vi "AddtoCurveList.vi"(8 "error in (no error)":errorcluster caption="entrée d'erreur (pas d'erreur)", 11 "Interface en entrée":refnum<class "Interface.lvclass"> caption="DNL_LabVIEW Object in") -> (0 "error out":errorcluster caption="sortie d'erreur", 3 "Interface en sortie":refnum<class "Interface.lvclass"> caption="DNL_LabVIEW Object out")   [LabVIEW 2010, in "Interface.lvclass"]
uses:
  Interface.lvclass
  Interface.lvclass/Interface.ctl
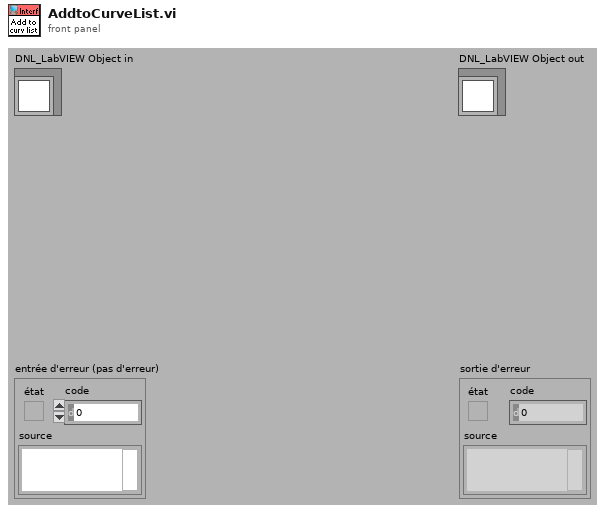
[diagram p1: front panel]
types:
  T1 = typedef "Interface.lvclass/CurveSetup.ctl" = cluster{"CurveName":string, "YParam":string, "XParam":string, "ZParam ":string, "GroupName":string, "LinWdth":u8, "PntCol":u32, "LinCol":u32, "LablFor":u8, "XScale":u32, "YScale":u32, "Interpol":u8, "DisplayName":string, "FillType":i16, "LineStyle":u8, "PntStyle":u8, "BarTyp":u8, "GraphIndex":i32, "Visible":bool, "XScaleName":string, "YScaleName":string, "XYGraph_Ref":refnum<vi>, "Data Only":bool, "DataQ Ref":refnum<queue>, "XParQ Ref":refnum<queue>, "XParamInd":i32}
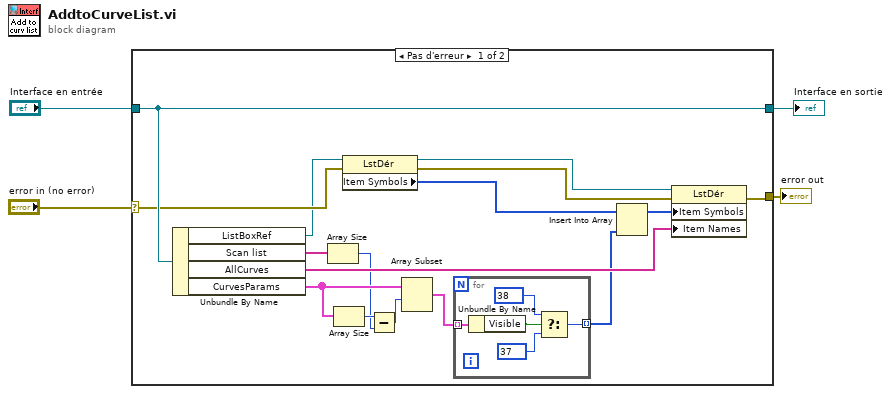
[diagram p0: block diagram]
diagram:
  n1 = case shown="Pas d'erreur" "error in (no error)" {
    selector: "error in (no error)" -> [w14 w27]
    tunnel: [w12 w27] -> w3
    tunnel: [w17 w26] -> w1
    tunnel: "Interface en entrée" -> [w17 w26]
    frame No Error {
      n2 = Unbundle By Name(w17) -> ("ListBoxRef"=w11:refnum<vi>, "Scan list"=w15:string[], "AllCurves"=w16:string[], "CurvesParams"=w10:T1[])
      n3 = Array Size(array=w15) -> (size(s)=w8:i32)
      n4 = Array Size(array=w10) -> (size(s)=w9:i32)
      n5 = property on="Nœud de propriété" class="LstDér"(reference=w11, error in=w14) -> (reference out=w18:refnum<vi>, error out=w13:errorcluster, "Item Symbols"=w19:i32[])
      n6 = Subtract(x=w9, y=w8) -> (x-y=w7:i32)
      n7 = Array Subset(array=w10, index=w7) -> (w5:T1[])  [unwired: 1 in]
      n8 = for {
        tunnel: [w22] -> w6 mode=indexing
        tunnel: w5 -> [w21] mode=indexing
        n9 = Unbundle By Name(w21) -> ("Visible"=w25:bool)
        n10 = Select(t=38, s=w25, f=37) -> (s? t:f=w22:i32)
      }
      n11 = Insert Into Array(array=w19, new element=w6) -> (w20:i32[])  [unwired: 1 in]
      n12 = property on="Nœud de propriété" class="LstDér"(reference=w18, error in=w13, "Item Symbols"=w20, "Item Names"=w16) -> (error out=w12:errorcluster)  [unwired: 1 out]
    }
    frame Error {
    }
  }
  "error out" <- w3
  "Interface en sortie" <- w1
